vi "Apply Gradient Cycler.vi"(8 "Reminder":dbl[](array[numeric]), 9 "Setpoint":dbl[](array[numeric]), 10 "Gradient":dbl[](array[numeric]) format="%#_13g", 11 "Iteration Interval":dbl=0.01 format="%#_13g") -> (3 "Array":dbl[](array[numeric]))   [LabVIEW 2023]
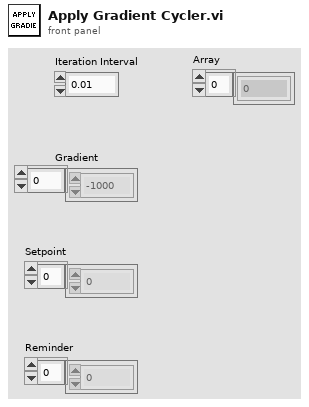
[diagram p1: front panel]
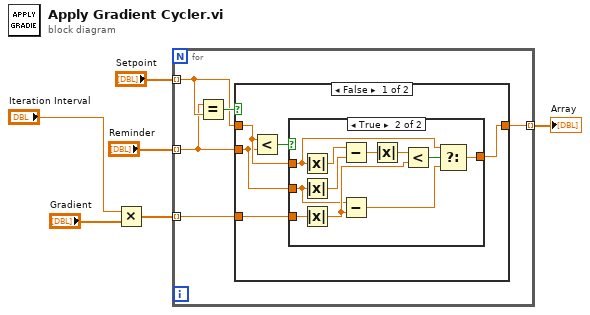
[diagram p0: block diagram]
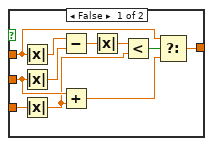
[diagram p2: hidden frame]
diagram:
  n1 = Multiply(x="Iteration Interval", y="Gradient") -> (x*y=w6:dbl[])
  n2 = for {
    tunnel: "Setpoint" -> [w10] mode=indexing
    tunnel: w6 -> [w7] mode=indexing
    tunnel: "Reminder" -> [w8] mode=indexing
    tunnel: [w9] -> w2 mode=indexing
    n3 = Equal?(x=w8, y=w10) -> (x = y?=w11:bool)
    n4 = case shown="False" w11 {
      tunnel: [w12 w39] -> w9
      tunnel: w10 -> [w15 w39]
      tunnel: w8 -> [w14 _]
      tunnel: w7 -> [w13 _]
      frame False {
        n5 = Less?(x=w15, y=w14) -> (x < y?=w16:bool)
        n6 = case shown="True" w16 {
          tunnel: w15 -> [w19 w29]
          tunnel: w14 -> [w22 w31]
          tunnel: w13 -> [w27 w38]
          tunnel: [w17 w28] -> w12
          frame False {
            n7 = Absolute Value(x=w19) -> (abs(x)=w25:dbl)
            n8 = Absolute Value(x=w22) -> (abs(x)=w26:dbl)
            n9 = Absolute Value(x=w27) -> (abs(x)=w21:dbl)
            n10 = Subtract(x=w25, y=w26) -> (x-y=w24:dbl)
            n11 = Add(x=w22, y=w21) -> (x+y=w20:dbl)
            n12 = Absolute Value(x=w24) -> (abs(x)=w23:dbl)
            n13 = Less?(x=w23, y=w21) -> (x < y?=w18:bool)
            n14 = Select(t=w19, s=w18, f=w20) -> (s? t:f=w17:dbl)
          }
          frame True {
            n15 = Absolute Value(x=w29) -> (abs(x)=w36:dbl)
            n16 = Absolute Value(x=w31) -> (abs(x)=w37:dbl)
            n17 = Absolute Value(x=w38) -> (abs(x)=w32:dbl)
            n18 = Subtract(x=w36, y=w37) -> (x-y=w35:dbl)
            n19 = Subtract(x=w31, y=w32) -> (x-y=w30:dbl)
            n20 = Absolute Value(x=w35) -> (abs(x)=w34:dbl)
            n21 = Less?(x=w34, y=w32) -> (x < y?=w33:bool)
            n22 = Select(t=w29, s=w33, f=w30) -> (s? t:f=w28:dbl)
          }
        }
      }
      frame True {
      }
    }
  }
  "Array" <- w2
